vi "Cycle_History_Logging.vi"(8 "error in (no error)":errorcluster, 11 "Diag Cycle String Out":string[][](array[string])) -> (0 "error out":errorcluster)   [LabVIEW 2021]
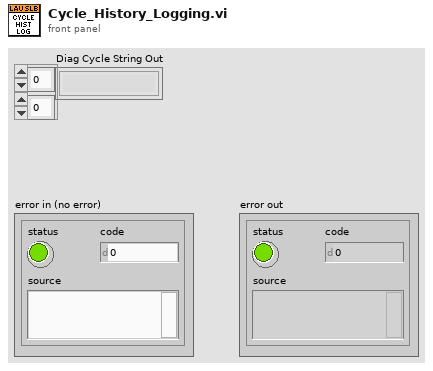
[diagram p1: front panel]
types:
  T1 = enum16{"open", "replace", "create", "open or create", "replace or create", "replace or create with confirmation"}
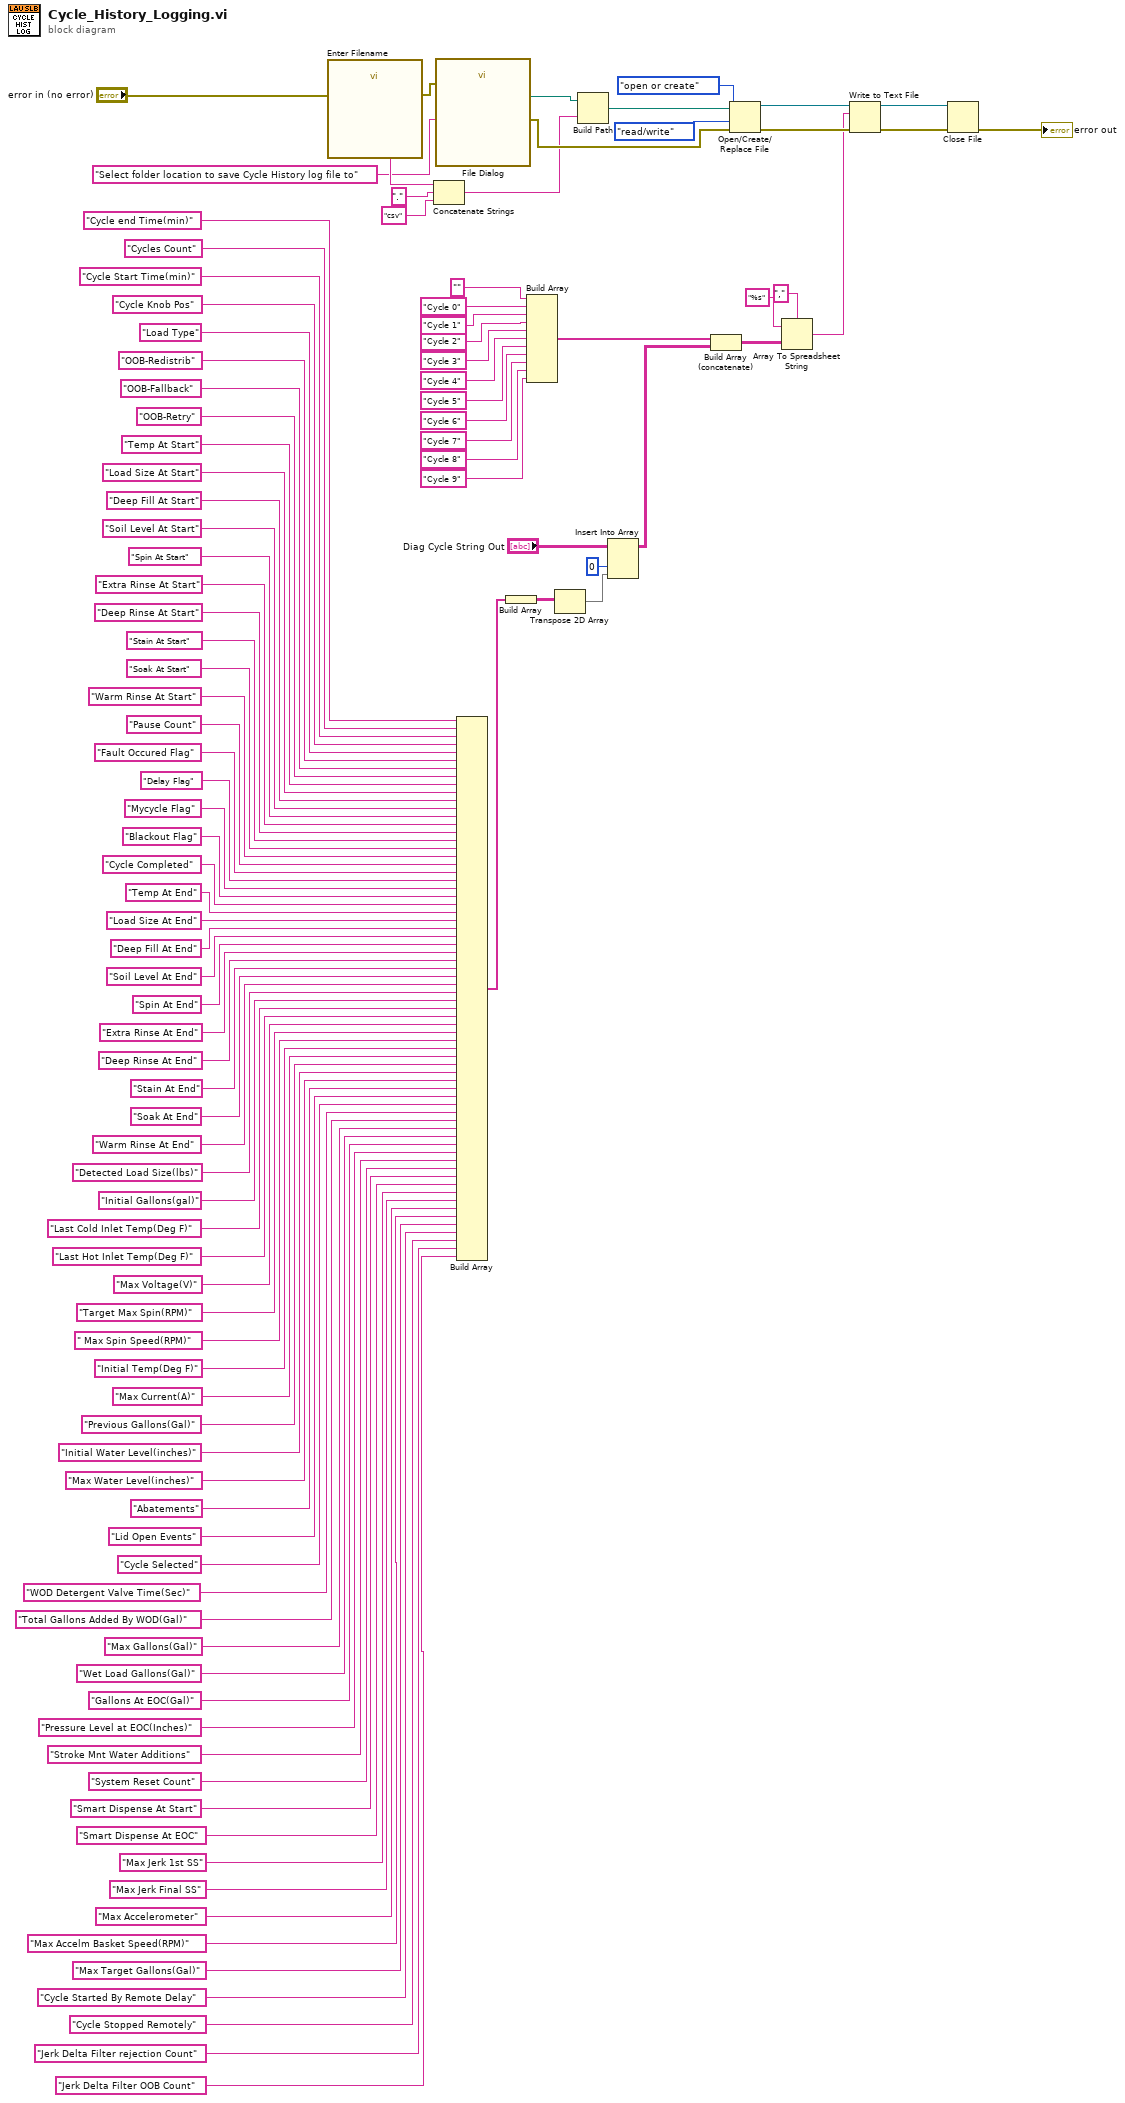
[diagram p0: block diagram]
diagram:
  n1 = call "Enter Filename"("error in (no error)"="error in (no error)") -> ("Filename"=w105:string, "error out"=w100:errorcluster)  [unwired: 16 in, 1 out]
  n2 = Concatenate Strings(w105, "." ("string"), "csv" ("string")) -> (w104:string)
  n3 = call "File Dialog"("prompt"="Select folder location to save Cycle History log file to", "error in"=w100) -> ("selected path"=w37:path, "error out"=w106:errorcluster)  [unwired: 10 in, 2 out]
  n4 = Build Array("Cycle end Time(min)" ("delimiter (\\t)"), "Cycles Count" ("delimiter (\\t)"), "Cycle Start Time(min)" ("delimiter (\\t)"), "Cycle Knob Pos" ("delimiter (\\t)"), "Load Type" ("delimiter (\\t)"), "OOB-Redistrib" ("delimiter (\\t)"), "OOB-Fallback" ("delimiter (\\t)"), "OOB-Retry" ("delimiter (\\t)"), "Temp At Start" ("delimiter (\\t)"), "Load Size At Start" ("delimiter (\\t)"), "Deep Fill At Start" ("delimiter (\\t)"), "Soil Level At Start" ("delimiter (\\t)"), "Spin At Start" ("delimiter (\\t)"), "Extra Rinse At Start" ("delimiter (\\t)"), "Deep Rinse At Start" ("delimiter (\\t)"), "Stain At Start" ("delimiter (\\t)"), "Soak At Start" ("delimiter (\\t)"), "Warm Rinse At Start" ("delimiter (\\t)"), "Pause Count" ("delimiter (\\t)"), "Fault Occured Flag" ("delimiter (\\t)"), "Delay Flag" ("delimiter (\\t)"), "Mycycle Flag" ("delimiter (\\t)"), "Blackout Flag" ("delimiter (\\t)"), "Cycle Completed" ("delimiter (\\t)"), "Temp At End" ("delimiter (\\t)"), "Load Size At End" ("delimiter (\\t)"), "Deep Fill At End" ("delimiter (\\t)"), "Soil Level At End" ("delimiter (\\t)"), "Spin At End" ("delimiter (\\t)"), "Extra Rinse At End" ("delimiter (\\t)"), "Deep Rinse At End" ("delimiter (\\t)"), "Stain At End" ("delimiter (\\t)"), "Soak At End" ("delimiter (\\t)"), "Warm Rinse At End" ("delimiter (\\t)"), "Detected Load Size(lbs)" ("delimiter (\\t)"), "Initial Gallons(gal)" ("delimiter (\\t)"), "Last Cold Inlet Temp(Deg F)" ("delimiter (\\t)"), "Last Hot Inlet Temp(Deg F)" ("delimiter (\\t)"), "Max Voltage(V)" ("delimiter (\\t)"), "Target Max Spin(RPM)" ("delimiter (\\t)"), " Max Spin Speed(RPM)" ("delimiter (\\t)"), "Initial Temp(Deg F)" ("delimiter (\\t)"), "Max Current(A)" ("delimiter (\\t)"), "Previous Gallons(Gal)" ("delimiter (\\t)"), "Initial Water Level(inches)" ("delimiter (\\t)"), "Max Water Level(inches)" ("delimiter (\\t)"), "Abatements" ("delimiter (\\t)"), "Lid Open Events" ("delimiter (\\t)"), "Cycle Selected" ("delimiter (\\t)"), "WOD Detergent Valve Time(Sec)" ("delimiter (\\t)"), "Total Gallons Added By WOD(Gal)" ("delimiter (\\t)"), "Max Gallons(Gal)" ("delimiter (\\t)"), "Wet Load Gallons(Gal)" ("delimiter (\\t)"), "Gallons At EOC(Gal)" ("delimiter (\\t)"), "Pressure Level at EOC(Inches)" ("delimiter (\\t)"), "Stroke Mnt Water Additions" ("delimiter (\\t)"), "System Reset Count" ("delimiter (\\t)"), "Smart Dispense At Start" ("delimiter (\\t)"), "Smart Dispense At EOC" ("delimiter (\\t)"), "Max Jerk 1st SS" ("delimiter (\\t)"), "Max Jerk Final SS" ("delimiter (\\t)"), "Max Accelerometer" ("delimiter (\\t)"), "Max Accelm Basket Speed(RPM)" ("delimiter (\\t)"), "Max Target Gallons(Gal)" ("delimiter (\\t)"), "Cycle Started By Remote Delay" ("delimiter (\\t)"), "Cycle Stopped Remotely" ("delimiter (\\t)"), "Jerk Delta Filter rejection Count" ("delimiter (\\t)"), "Jerk Delta Filter OOB Count" ("delimiter (\\t)")) -> (w29:string[])
  n5 = Build Array(w29) -> (w28:string[][])
  n6 = Build Array("" ("delimiter (\\t)"), "Cycle 0" ("delimiter (\\t)"), "Cycle 1" ("delimiter (\\t)"), "Cycle 2" ("delimiter (\\t)"), "Cycle 3" ("delimiter (\\t)"), "Cycle 4" ("delimiter (\\t)"), "Cycle 5" ("delimiter (\\t)"), "Cycle 6" ("delimiter (\\t)"), "Cycle 7" ("delimiter (\\t)"), "Cycle 8" ("delimiter (\\t)"), "Cycle 9" ("delimiter (\\t)")) -> (w32:string[])
  n7 = Transpose 2D Array(2D array=w28) -> (transposed array=w22:string[][])
  n8 = Build Path(base path=w37, name or relative path=w104) -> (appended path=w86:path)
  n9 = Insert Into Array(array="Diag Cycle String Out", index (col)=0 ("disabled index (col)"), new element=w22) -> (w23:string[][])  [unwired: 1 in]
  n10 = Build Array (concatenate)(w32, w23) -> (w31:string[][])
  n11 = Open/Create/Replace File(file path (use dialog)=w86, error in=w106, operation (0:open)=T1."open or create", access (0:read/write)=enum16{"read/write", "read-only", "write-only"}."read/write") -> (refnum out=w36:refnum<file>, error out=w35:errorcluster)  [unwired: 2 in, 1 out]
  n12 = Array To Spreadsheet String(delimiter (Tab)=",", array=w31, 3:"%s" ("format string")) -> (spreadsheet string=w30:string)
  n13 = Write to Text File(file (use dialog)=w36, text=w30, error in=w35) -> (refnum out=w27:refnum<file>, error out=w26:errorcluster)  [unwired: 1 in, 1 out]
  n14 = Close File(refnum=w27, error in=w26) -> (error out=→"error out":errorcluster)  [unwired: 1 out]
